vi "Generate Documentation--dialog.vi"(8 "error in":errorcluster, 11 "Project Path":path) -> (0 "error out":errorcluster)   [LabVIEW 2019, in "Panther Dashboard.lvlib"]
doc: "<b>Note:</b> This VI was modified by the <b>Validate DQMH Module</b> tool to turn off automatic error handling."
uses:
  Panther Dashboard.lvlib
  <vilib>/Wovalab/AntiDoc/Document Type/Add-ons/LabVIEW Project/Lv Proj/Lv Proj.lvclass
  C:/Program Files (x86)/National Instruments/LabVIEW 2019/vi.lib/Wovalab/AntiDoc/Document Type/Document/Document Type.lvclass
  <vilib>/Utility/miscctls.llb/LVPointTypeDef.ctl
  <vilib>/Wovalab/AntiDoc/Document Type/Add-ons/LabVIEW Project/Lv Proj Config/Lv Proj Config.lvclass
  C:/Program Files (x86)/National Instruments/LabVIEW 2019/vi.lib/Wovalab/AntiDoc/Document Type/Config/Config.lvclass
  <vilib>/Wovalab/AntiDoc/Document Type/Document/Document Type.lvclass/Document Type.ctl
  <vilib>/Wovalab/AntiDoc/Document Type/Add-ons/LabVIEW Project/Lv Proj Config/Lv Proj Config.lvclass/Lv Proj Config.ctl
  <vilib>/Wovalab/AntiDoc/Doc/Author Info--cluster.ctl
  <vilib>/Wovalab/AntiDoc/Doc/Doc.lvclass/Doc.ctl
  <vilib>/Wovalab/AntiDoc/Document Type/Document/Read Config.vi
  <vilib>/Wovalab/AntiDoc/Document Type/Add-ons/LabVIEW Project/Lv Proj Config/Write Project Path.vi
  <vilib>/Wovalab/AntiDoc/Document Type/Document/Write Config.vi
  <vilib>/Wovalab/AntiDoc/Doc/Write Document File Name.vi
  <vilib>/Wovalab/AntiDoc/Doc/Write Documentation Folder.vi
  <vilib>/Wovalab/AntiDoc/Document Type/Config/Config.lvclass
  <vilib>/Wovalab/AntiDoc/Progress Bar/Progress Bar.lvlib
  <vilib>/Wovalab/AntiDoc/Document Type/Document/Document Type.lvclass
  <vilib>/Wovalab/AntiDoc/Doc/Doc.lvclass
panel:
  in  "Open the document at the end of the generation":bool=TRUE
  in  "Generate":bool
  out "Progress Bar":u8(slide) caption="Waiting for user action..." max=100 scale=0.0..100.0
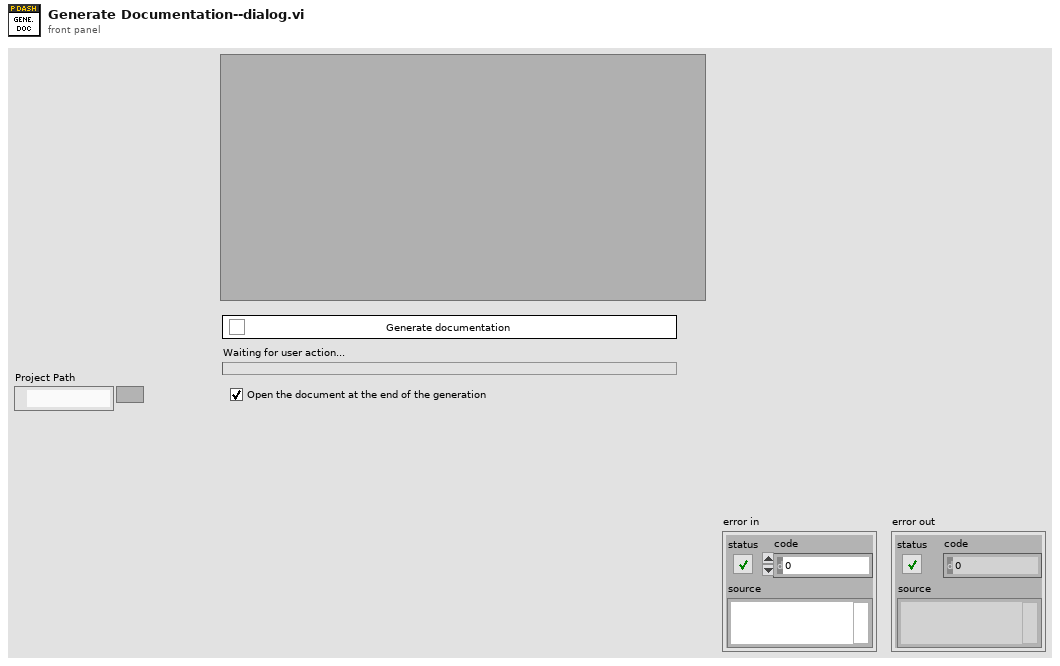
[diagram p1: front panel]
types:
  T1 = enum32{"Invalid", "Standard", "Closed", "Hidden", "Minimized", "Maximized"}
  T2 = typedef "LVPointTypeDef.ctl" = cluster{"Horizontal":i16, "Vertical":i16}
  T3 = typedef "AntiDoc.lvlib/Doc.lvclass/Author Info--cluster.ctl" = cluster{"Name":string, "Email":string}
  T4 = typedef "AntiDoc.lvlib/Document Type.lvclass/Final Documentation Info--cluster.ctl" = cluster{"Title":string, "Author Name":string, "Author Email":string, "Destination Folder":path, "File Name":string}
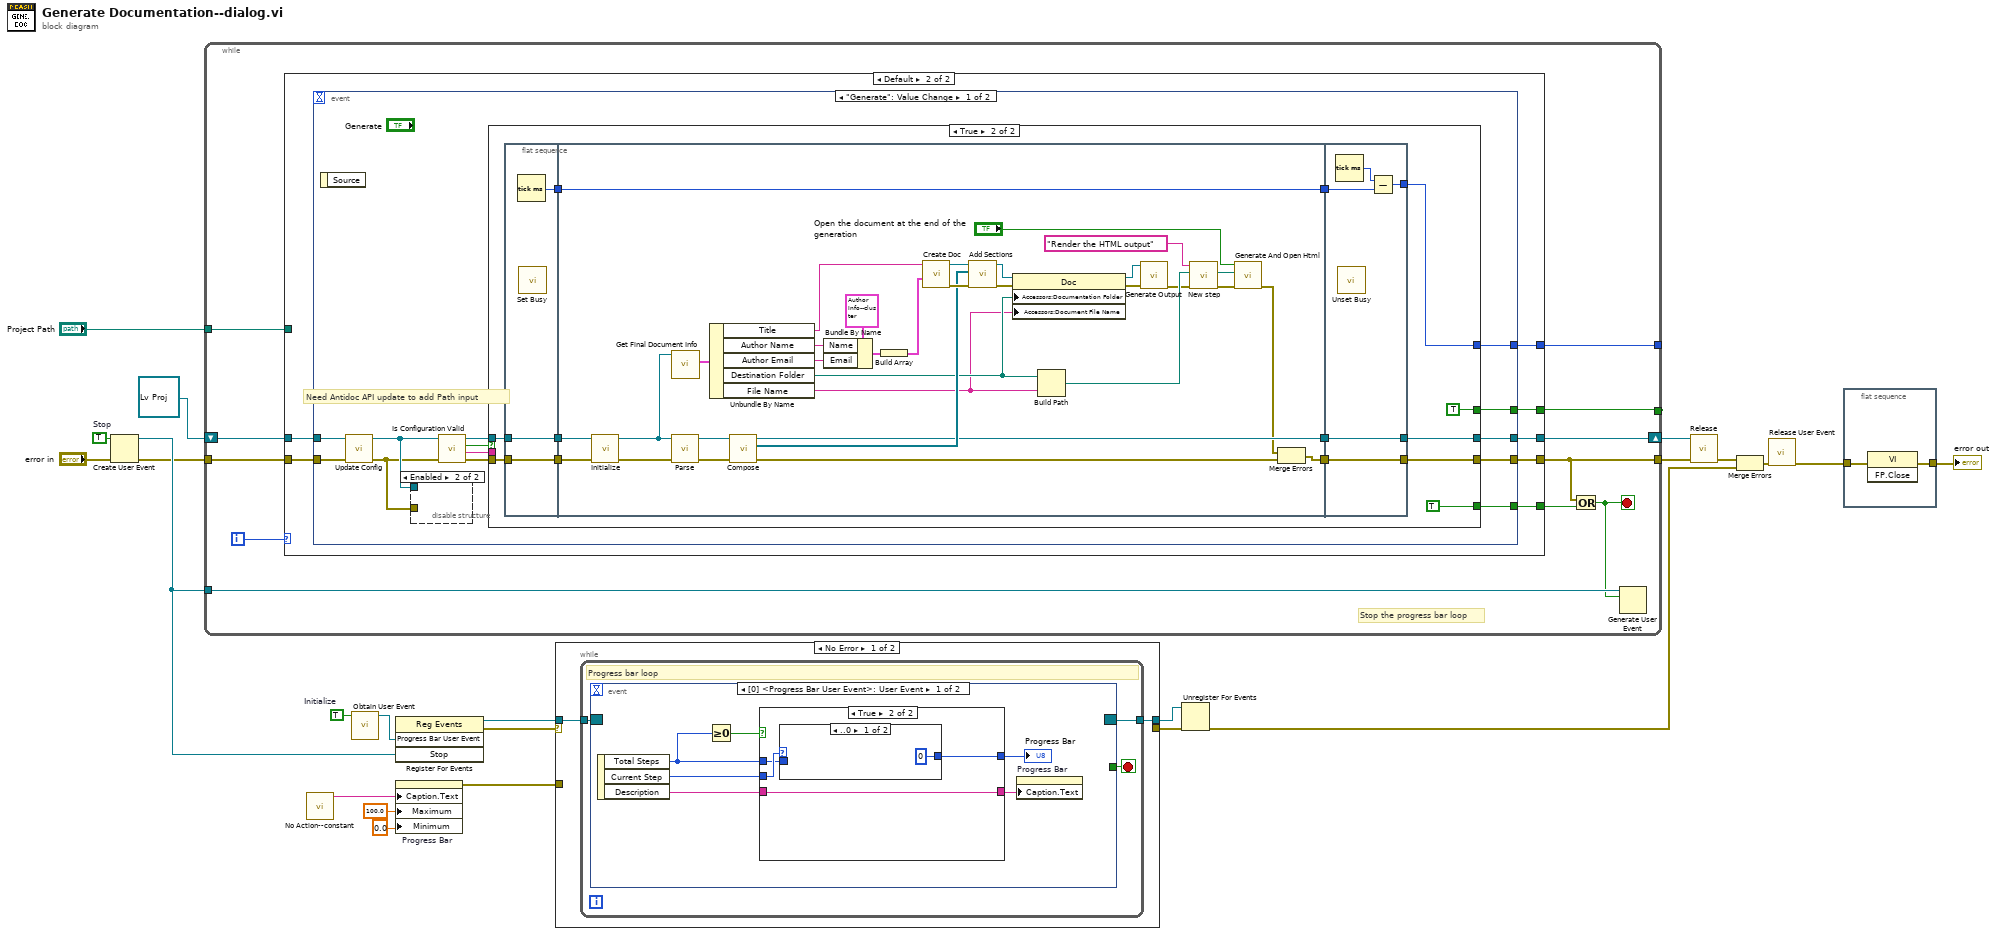
[diagram p0: block diagram]
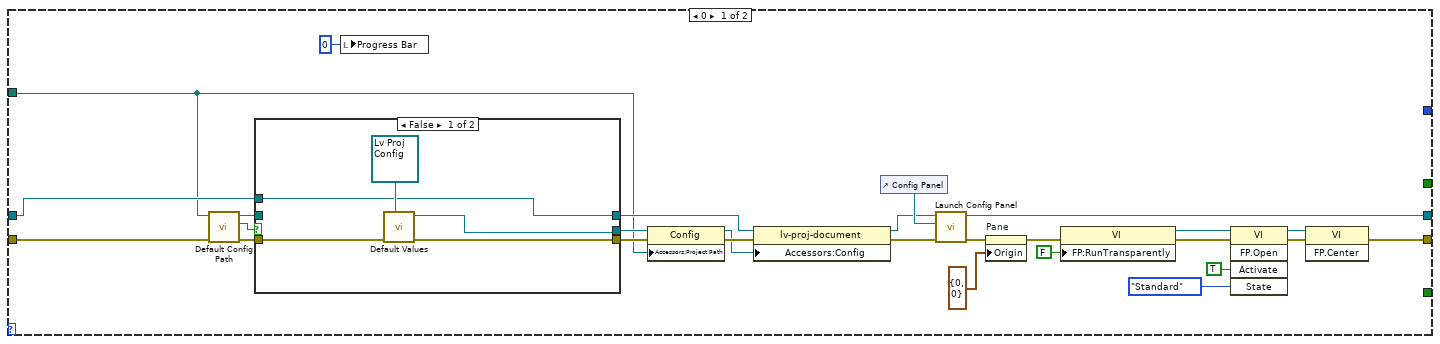
[diagram p2: hidden frame]
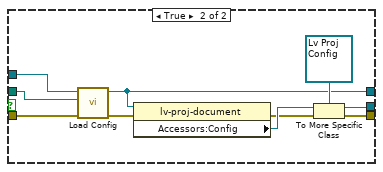
[diagram p3: hidden frame]
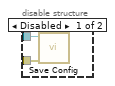
[diagram p4: hidden frame]
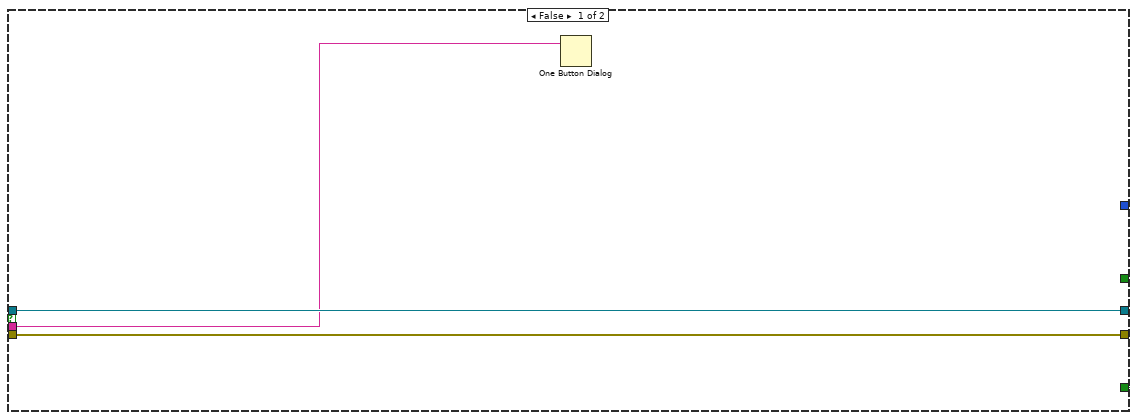
[diagram p5: hidden frame]
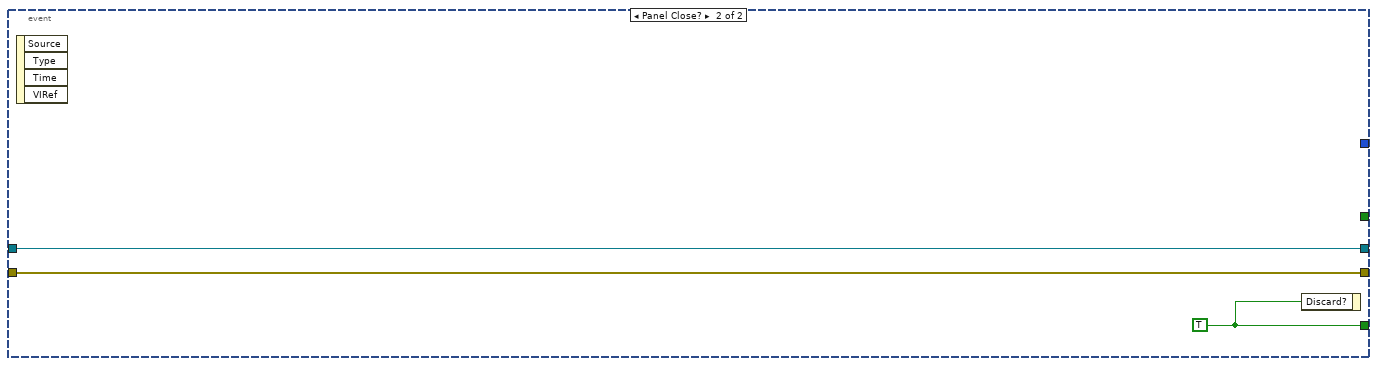
[diagram p6: hidden frame]
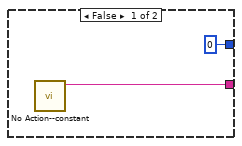
[diagram p7: hidden frame]
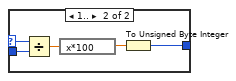
[diagram p8: hidden frame]
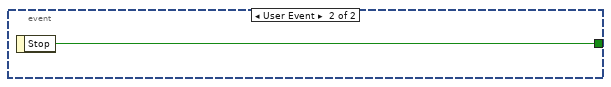
[diagram p9: hidden frame]
diagram:
  w13 = TRUE  # Initialize
  w23 = TRUE  # Stop
  n1 = Create User Event(user event datatype=w23, error in="error in") -> (user event=w12:refnum<user-event>, error out=w11:errorcluster)
  n2 = while {
    tunnel: [w27] -> w6
    tunnel: w12 -> [w34]
    tunnel: [w32] -> _
    tunnel: [w31] -> _
    shift-right: [w29] -> w7
    shift-left: refnum<class "Lv Proj.lvclass"> refnum ("Lv Proj Document Type.lvlib:lv-proj-document") -> [w33]
    tunnel: w11 -> [w28]
    tunnel: "Project Path" -> [w24]
    i -> [w30]
    stop <- w26 stop-if-true
    # "Stop the progress bar loop"
    n3 = case shown="Default" w30 {
      tunnel: [w55 w83] -> w27
      tunnel: [_ w82] -> w25
      tunnel: w33 -> [w41 w81]
      tunnel: [_ w80] -> w32
      tunnel: [w49 w79] -> w29
      tunnel: [_ w78] -> w31
      tunnel: w28 -> [w38 w77]
      tunnel: w24 -> [w40 _]
      frame 0 {
        n4 = call "Default Config Path.vi"("error in"=w38, "Project Path"=w40) -> ("error out"=w39:errorcluster, "File Exists?"=w37:bool, "Config Path"=w36:path)  [unwired: 7 in]
        n5 = case shown="False" w37 {
          tunnel: [w64 w75] -> w48
          tunnel: [w65 w72] -> w47
          tunnel: [w62 w70] -> w42
          tunnel: w41 -> [w62 w69]
          tunnel: w39 -> [w66 w68]
          tunnel: w36 -> [_ w67]
          frame False {
            n6 = call-dynamic "Default Values.vi"("Type"=refnum<class "Lv Proj Config.lvclass"> refnum ("Lv Proj Document Type.lvlib:Config"), "error in"=w66) -> ("error out"=w65:errorcluster, "Config out"=w64:refnum<class "Lv Proj Config.lvclass">)  [unwired: 8 in]
          }
          frame True {
            n7 = call <vilib>:"Load Config.vi"("error in"=w68, "File Path"=w67, "Document in"=w69) -> ("error out"=w71:errorcluster, "Document out"=w70:refnum<class "Lv Proj.lvclass">)  [unwired: 7 in]
            n8 = property class="lv-proj-document"(reference=w70, error in=w71) -> (error out=w73:errorcluster, "Accessors:Config"=w76:refnum<class "Config.lvclass">)  [unwired: 1 out]
            n9 = To More Specific Class(target class=refnum<class "Lv Proj Config.lvclass"> refnum ("Lv Proj Document Type.lvlib:Config"), reference=w76, error in=w73) -> (specific class reference=w75:refnum<class "Lv Proj Config.lvclass">, error out=w72:errorcluster)
          }
        }
        n10 = local write "Progress Bar"(u8 0 ("Progress Bar")) -> ()
        n11 = property class="Config"(reference=w48, error in=w47, "Accessors:Project Path"=w40) -> (reference out=w44:refnum<class "Lv Proj Config.lvclass">, error out=w46:errorcluster)
        n12 = property class="lv-proj-document"(reference=w42, error in=w46, "Accessors:Config"=w44) -> (reference out=w43:refnum<class "Lv Proj.lvclass">, error out=w45:errorcluster)
        n13 = control-ref of="Config Panel"() -> (w50:refnum<vi>)
        n14 = call <vilib>:"Launch Config Panel.vi"("error in"=w45, "Sub Panel"=w50, "Document in"=w43) -> ("error out"=w60:errorcluster, "Document out"=w49:refnum<class "Lv Proj.lvclass">)  [unwired: 7 in]
        n15 = property on="Pane" class="Pane"(error in=w60, "Origin"=T2 {"Horizontal"=0, "Vertical"=0}) -> (error out=w54:errorcluster)  [unwired: 1 in, 1 out]
        n16 = property class="VI"(error in=w54, "FP:RunTransparently"=FALSE ("Front Panel Window:Run VI Transparently")) -> (reference out=w51:refnum<vi>, error out=w53:errorcluster)  [unwired: 1 in]
        n17 = invoke class="VI" method="FP.Open"(reference=w51, error in=w53, "Activate"=TRUE ("Activate?"), "State"=T1."Standard") -> (reference out=w58:refnum<vi>, error out=w59:errorcluster)  [unwired: 1 in, 3 out]
        n18 = invoke class="VI" method="FP.Center"(reference=w58, error in=w59) -> (error out=w55:errorcluster)  [unwired: 1 in, 2 out]
      }
      frame Default {
        n19 = event shown="[0] \"Generate\": Value Change" {
          selector: _ -> [_ _]
          dyn-events: _ -> [_ _]
          timeout: _ -> [_ _]
          tunnel: [w96 w156] -> w83
          tunnel: [w95 w158] -> w82
          tunnel: w81 -> [w91 w157]
          tunnel: [w93 _] -> w80
          tunnel: [w92 w157] -> w79
          tunnel: [w90 _] -> w78
          tunnel: w77 -> [w88 w156]
          event "Generate": Value Change {
            # "Need Antidoc API update to add Path input"
            n20 = event-data() -> ()  [unwired: 1 in, 1 out]
            n21 = call <vilib>:"Update Config.vi"("error in"=w88, "Document in"=w91) -> ("error out"=w84:errorcluster, "Document out"=w85:refnum<class "Lv Proj.lvclass">)  [unwired: 8 in]
            n22 = disable-structure shown="Enabled" {
              disable-tunnel: w85 -> [w98 _]
              disable-tunnel: w84 -> [w97 _]
              frame Disabled {
                n23 = call <vilib>:"Save Config.vi"("error in"=w97, "Document in"=w98) -> ()  [unwired: 9 in, 1 out]
              }
              frame Enabled {
              }
            }
            n24 = call-dynamic "Is Configuration Valid.vi"("error in"=w84, "Document in"=w85) -> ("error out"=w87:errorcluster, "Details"=w89:string, "Valid?"=w94:bool, "Document out"=w86:refnum<class "Lv Proj.lvclass">)  [unwired: 6 in]
            n25 = case shown="True" w94 {
              tunnel: [w99 w114] -> w96
              tunnel: [FALSE TRUE ("event data")] -> w95
              tunnel: w86 -> [w101 w109]
              tunnel: [_ w108] -> w93
              tunnel: [w101 w104] -> w92
              tunnel: [_ TRUE] -> w90
              tunnel: w89 -> [w100 _]
              tunnel: w87 -> [w99 w105]
              frame False {
                n26 = One Button Dialog(message=w100) -> ()  [unwired: 1 in, 1 out]
              }
              frame True {
                n27 = flat-sequence {
                  tunnel: [w118] -> w111
                  tunnel: [w117] -> w110
                  tunnel: w109 -> [w117]
                  tunnel: [w116] -> w106
                  tunnel: w105 -> [w116]
                  tunnel: [w136] -> w115
                  tunnel: [w141] -> w112
                  tunnel: w111 -> [w141]
                  tunnel: w110 -> [w137]
                  tunnel: w106 -> [w135]
                  tunnel: [w125] -> w103
                  tunnel: [w155] -> w114
                  tunnel: w115 -> [w155]
                  tunnel: w112 -> [w153]
                  tunnel: [w152] -> w108
                  tunnel: [w151] -> w104
                  tunnel: w103 -> [w151]
                  frame #0 {
                    n28 = Tick Count (ms)() -> (millisecond timer value=w118:u32)
                    n29 = call <vilib>:"Set Busy.vi"() -> ()  [unwired: 10 in, 2 out]
                  }
                  frame #1 {
                    n30 = call-dynamic "Initialize.vi"("error in"=w135, "Document in"=w137) -> ("error out"=w134:errorcluster, "Document out"=w133:refnum<class "Lv Proj.lvclass">)  [unwired: 8 in]
                    n31 = call-dynamic "Parse.vi"("error in"=w134, "Document in"=w133) -> ("error out"=w139:errorcluster, "Document out"=w140:refnum<class "Lv Proj.lvclass">)  [unwired: 8 in]
                    n32 = call-dynamic "Get Final Document Info.vi"("Document in"=w133) -> ("Final Documentation Info"=w132:T4)  [unwired: 9 in, 1 out]
                    n33 = Unbundle By Name(w132) -> ("Title"=w131:string, "Author Name"=w130:string, "Author Email"=w129:string, "Destination Folder"=w128:path, "File Name"=w127:string)
                    n34 = call-dynamic "Compose.vi"("error in"=w139, "Document in"=w140) -> ("error out"=w126:errorcluster, "Sections"=w138:refnum<class "Section.lvclass">[], "Document out"=w125:refnum<class "Lv Proj.lvclass">)  [unwired: 7 in]
                    n35 = Bundle By Name(cluster=T3 {"Name"="Wovalab", "Email"="contact@wovalab.com"} ("Author Info"), "Name"=w130, "Email"=w129) -> (w143:T3)
                    n36 = Build Array(w143) -> (w142:T3[])
                    n37 = call <vilib>:"Create Doc.vi"("Authors"=w142, "Title"=w131) -> ("error out"=w150:errorcluster, "Doc out"=w147:refnum<class "Doc.lvclass">)  [unwired: 8 in]
                    n38 = call <vilib>:"Add Sections.vi"("error in (no error)"=w150, "Sections"=w138, "Doc in"=w147) -> ("error out"=w149:errorcluster, "Doc out"=w146:refnum<class "Doc.lvclass">)  [unwired: 7 in]
                    n39 = property class="Doc"(reference=w146, error in=w149, "Accessors:Documentation Folder"=w128, "Accessors:Document File Name"=w127) -> (reference out=w145:refnum<class "Doc.lvclass">, error out=w148:errorcluster)
                    n40 = Build Path(base path=w128, name or relative path=w127) -> (appended path=w123:path)
                    n41 = call <vilib>:"Generate Output.vi"("error in"=w148, "Doc in"=w145) -> ("error out"=w121:errorcluster)  [unwired: 8 in, 1 out]
                    n42 = call <vilib>:"New step.vi"("error in"=w121, "Description"="Render the HTML output") -> ("error out"=w120:errorcluster)  [unwired: 9 in]
                    n43 = call "Generate And Open Html.vi"("error in"=w120, "Generated File Path"=w123, "Open Generated Document"="Open the document at the end of the generation") -> ("error out"=w124:errorcluster)  [unwired: 8 in]
                    n44 = Merge Errors(w124, w126) -> (w136:errorcluster)
                  }
                  frame #2 {
                    n45 = Tick Count (ms)() -> (millisecond timer value=w154:u32)
                    n46 = call <vilib>:"Unset Busy.vi"() -> ()  [unwired: 11 in, 1 out]
                    n47 = Subtract(x=w154, y=w153) -> (x-y=w152:u32)
                  }
                }
              }
            }
          }
          event Panel Close? {
            w158 = TRUE
            n48 = event-data() -> ()  [unwired: 1 in, 4 out]
            n49 = event-data("Discard?"=w158) -> ()  [unwired: 1 in, 1 out]
          }
        }
      }
    }
    n50 = Or(x=w27, y=w25) -> (x .or. y?=w26:bool)
    n51 = Generate User Event(user event=w34, event data cluster=w26) -> ()  [unwired: 2 in, 2 out]
  }
  n52 = call <vilib>:"No Action--constant.vi"() -> ("No Action"=w20:string)  [unwired: 11 in]
  n53 = call <vilib>:"Obtain User Event.vi"("Initialize(F)"=w13) -> ("Progress Bar User Event"=w14:refnum<user-event>)  [unwired: 10 in]
  n54 = register-events(w14, w12) -> (reference out=w15:refnum<event-registration>, error out=w16:errorcluster)  [unwired: 2 in]
  n55 = property on="Progress Bar" class="Slide (strict)"("Caption.Text"=w20, "Maximum"=100.0 ("Data Entry Limits:Maximum"), "Minimum"=0.0 ("Data Entry Limits:Minimum")) -> (error out=w19:errorcluster)  [unwired: 2 in, 1 out]
  n56 = case shown="No Error" w16 {
    selector: w16 -> [_ w183]
    tunnel: w15 -> [w160 w184]
    tunnel: [w159 w184] -> w17
    tunnel: [_ w183] -> w18
    tunnel: w19 -> [_ _]
    frame No Error {
      n57 = while {
        tunnel: w160 -> [w163]
        tunnel: [w161] -> w159
        stop <- w162 stop-if-true
        # "Progress bar loop"
        n58 = event shown="[0] <Progress Bar User Event>: User Event" {
          selector: w163 -> [_ _]
          dyn-events: [_ _] -> w161
          timeout: _ -> [_ _]
          tunnel: [_ w182] -> w162
          event User Event {
            n59 = event-data() -> ("Total Steps"=w166:i32, "Current Step"=w167:i32, "Description"=w168:string)  [unwired: 1 in]
            n60 = Greater Or Equal To 0?(x=w166) -> (x >= 0?=w169:bool)
            n61 = case shown="True" w169 {
              tunnel: w168 -> [_ w172]
              tunnel: w167 -> [_ w175]
              tunnel: w166 -> [_ w174]
              tunnel: [u8 0 w173] -> w165
              tunnel: [w171 w172] -> w164
              frame False {
                n62 = call <vilib>:"No Action--constant.vi"() -> ("No Action"=w171:string)  [unwired: 11 in]
              }
              frame True {
                n63 = case shown="..0" w175 {
                  selector: w175 -> [_ w181]
                  tunnel: w174 -> [_ w180]
                  tunnel: [u8 0 w177] -> w173
                  frame ..0 {
                  }
                  frame 1.. {
                    n64 = Divide(x=w181, y=w180) -> (x/y=w178:dbl)
                    n65 = expression code="x*100"(w178) -> (w179:dbl)
                    n66 = To Unsigned Byte Integer(number=w179) -> (unsigned 8bit integer=w177:u8)
                  }
                }
              }
            }
            "Progress Bar" <- w165
            n67 = property on="Progress Bar" class="Slide (strict)"("Caption.Text"=w164) -> ()  [unwired: 2 in, 2 out]
          }
          event User Event {
            n68 = event-data() -> ("Stop"=w182:bool)  [unwired: 1 in]
          }
        }
      }
    }
    frame Error {
    }
  }
  n69 = Unregister For Events(event registration refnum=w17, error in=w18) -> (error out=w9:errorcluster)
  n70 = call-dynamic "Release.vi"("error in"=w6, "Document in"=w7) -> ("error out"=w5:errorcluster)  [unwired: 9 in]
  n71 = Merge Errors(w5, w9) -> (w8:errorcluster)
  n72 = call <vilib>:"Release User Event.vi"("error in"=w8) -> ("error out"=w3:errorcluster)  [unwired: 10 in]
  n73 = flat-sequence {
    tunnel: w3 -> [w186]
    tunnel: [w185] -> w2
    frame #0 {
      n74 = invoke class="VI" method="FP.Close"(error in=w186) -> (error out=w185:errorcluster)  [unwired: 2 in, 2 out]
    }
  }
  "error out" <- w2
